vi "Pose3d_RelativeTo.vi"(9 "other Pose3d":T1={"Translation3d"={"X"=0.0, "Y"=0.0, "Z"=0.0}, "Rotation3d"={"Q_quaternion"={"R"=1.0, "V"=[0.0, 0.0, 0.0]}}} {"Translation3d"."Z" format="%14.3f"; "Translation3d"."Y" format="%14.3f"; "Translation3d"."X" format="%14.3f"}, 11 "in Pose3d":T1={"Translation3d"={"X"=0.0, "Y"=0.0, "Z"=0.0}, "Rotation3d"={"Q_quaternion"={"R"=1.0, "V"=[0.0, 0.0, 0.0]}}} {"Translation3d"."Z" format="%14.3f"; "Translation3d"."Y" format="%14.3f"; "Translation3d"."X" format="%14.3f"}) -> (3 "out Pose3d":T1={"Translation3d"={"X"=0.0, "Y"=0.0, "Z"=0.0}, "Rotation3d"={"Q_quaternion"={"R"=1.0, "V"=[0.0, 0.0, 0.0]}}} {"Translation3d"."Z" format="%14.3f"; "Translation3d"."Y" format="%14.3f"; "Translation3d"."X" format="%14.3f"})   [LabVIEW 2019, in "Trajectory_Library.lvlib"]
doc: "Returns the other pose relative to the current pose.\n\nThis function can often be used for trajectory tracking or pose stabilization algorithms to get the error between the reference and the current pose.\n\nParameters:\n - IN POSE3D - The POSE data structure\n - OTHER POSE3D - The pose that is the origin of the new coordinate frame that the current pose will be converted into.\n\nReturn:\n - OUT POSE3D - The current pose relative to the new origin pose."
uses:
  Trajectory_Library.lvlib
  POSE3D.ctl
  TRANSLATION3D.ctl
  ROTATION3D.ctl
  QUATERNION.ctl
  Transform3d_Create_Trans3dRot3d.vi
  Translation3d_Minus.vi
  Translation3d_RotateBy.vi
  Rotation3d_UnaryMinus.vi
  Pose3d_getTranslation3d.vi
  Pose3d_getRotation3d.vi
  Rotation3d_Minus.vi
  Translation3d_Create.vi
  Rotation3d_GetQuaterion.vi
  Quaternion_New.vi
  Quaternion_Times.vi
  Quaternion_Inverse.vi
  Quaternion_Get_All.vi
  Rotation3d_Create_Quaternion.vi
  Rotation3d_RotateBy.vi
  Quaternion_Normalize.vi
  Quaternion_New_Default.vi
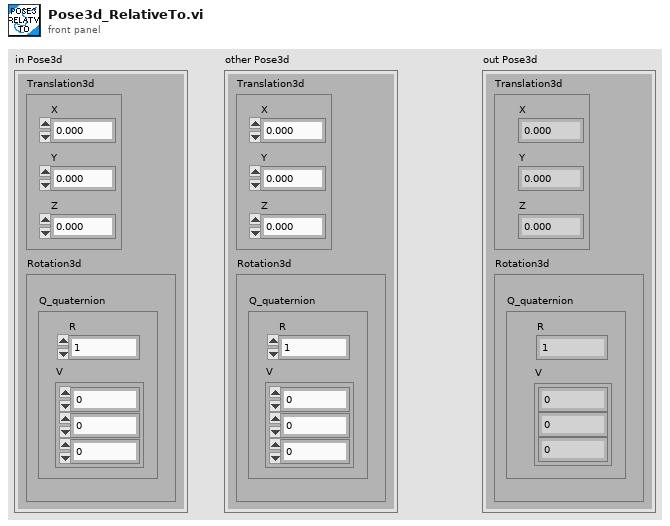
[diagram p1: front panel]
types:
  T1 = typedef "Trajectory_Library.lvlib/POSE3D.ctl" = cluster{"Translation3d":T2, "Rotation3d":T3}
  T2 = typedef "Trajectory_Library.lvlib/TRANSLATION3D.ctl" = cluster{"X":dbl, "Y":dbl, "Z":dbl}
  T3 = typedef "Trajectory_Library.lvlib/ROTATION3D.ctl" = cluster{"Q_quaternion":T4}
  T4 = typedef "Trajectory_Library.lvlib/QUATERNION.ctl" = cluster{"R":dbl, "V":dbl[]}
  T5 = typedef "Trajectory_Library.lvlib/TRANSFORM3D.ctl" = cluster{"TRANSLATION3D":T2, "ROTATION3D":T3, "XF":bool}
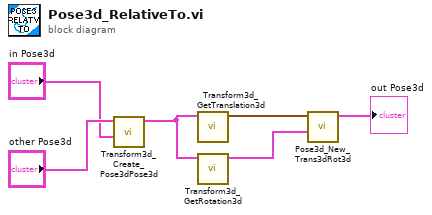
[diagram p0: block diagram]
diagram:
  n1 = call "Transform3d_Create_Pose3dPose3d.vi"("last Pose3d"="in Pose3d", "initial Pose3d"="other Pose3d") -> ("Transform3d"=w3:T5)  [unwired: 9 in]
  n2 = call "Transform3d_GetTranslation3d.vi"("in Transform3d"=w3) -> ("Translation3d"=w1:T2)  [unwired: 10 in]
  n3 = call "Transform3d_GetRotation3d.vi"("in Transform3d"=w3) -> ("Rotation3d"=w2:T3)  [unwired: 10 in]
  n4 = call "Pose3d_New_Trans3dRot3d.vi"("Rotation3d"=w2, "Translation3d"=w1) -> ("outPose3d"=→"out Pose3d":T1)  [unwired: 9 in]
